vi "Control Enable Disable.vi"(0 "Control References":refnum<vi>[](array[refnum]), 5 "Disable?":bool, 11 "Error In":errorcluster) -> (15 "Error Out":errorcluster)   [LabVIEW 2023, in "File and Path Operations.lvlib"]
doc: "This VI takes an array of control/indicator references and a Boolean input to enable or disable and grey out the referenced controls."
uses:
  File and Path Operations.lvlib
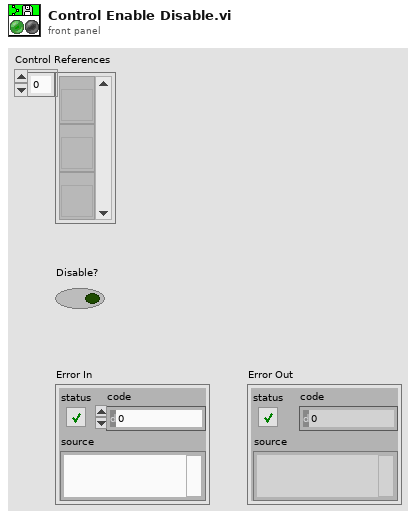
[diagram p1: front panel]
types:
  T1 = enum8{"Enabled", "Disabled", "Disabled and Grayed Out"}
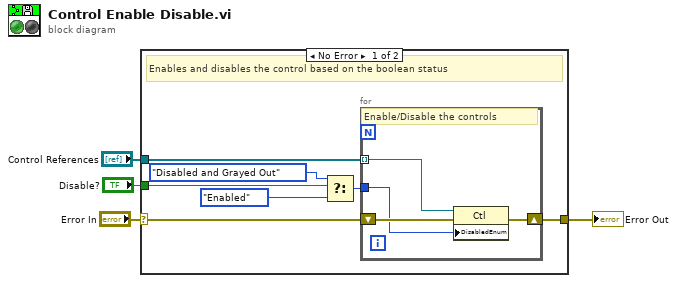
[diagram p0: block diagram]
diagram:
  n1 = case shown="No Error" "Error In" {
    selector: "Error In" -> [w11 w16]
    tunnel: "Control References" -> [w9 _]
    tunnel: [w10 w16] -> w1
    tunnel: "Disable?" -> [w8 _]
    frame No Error {
      # "Enables and disables the control based on the boolean status"
      n2 = Select(t=T1."Disabled and Grayed Out" ("Disabled"), s=w8, f=T1."Enabled" ("Disabled")) -> (s? t:f=w7:T1)
      n3 = for {
        shift-right: [w14] -> w10
        shift-left: w11 -> [w15]
        tunnel: w9 -> [w13] mode=indexing
        tunnel: w7 -> [w12]
        # "Enable/Disable the controls"
        n4 = property class="Ctl"(reference=w13, error in=w15, "DisabledEnum"=w12) -> (error out=w14:errorcluster)  [unwired: 1 out]
      }
    }
    frame Error {
    }
  }
  "Error Out" <- w1
